vi "Event 練習-五子棋-介面.vi"() -> ()   [LabVIEW 2019, in "Event 2-上課練習.lvlib"]
uses:
  <vilib>/Utility/miscctls.llb/LVPoint32TypeDef.ctl
panel:
  out "Coords":T1
  out "黑子":T2[][](array[typedef])
  out "白子":T3[][](array[typedef])
  in  "stop":bool
  # "五子棋程式-1（練習Event搭配State Machine的結構)\n1. 練習如何建立棋盤、黑子、白子；\n2. 按下「半黑白」可產生上下各一半的棋子，再按一次清除；\n3. 在滑鼠按下處，產生黑子；再按一次可以消除；"
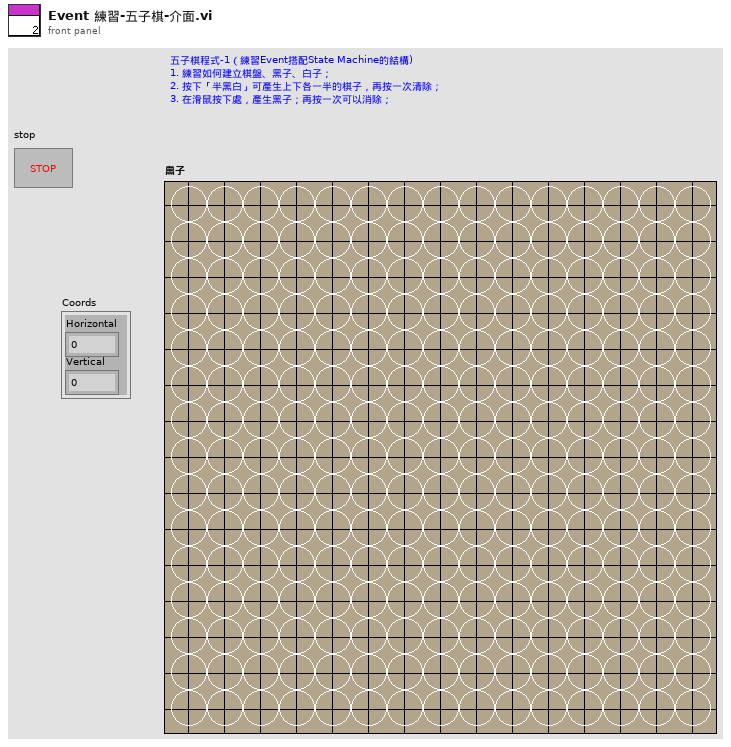
[diagram p1: front panel]
types:
  T1 = typedef "LVPoint32TypeDef.ctl" = cluster{"Horizontal":i32, "Vertical":i32}
  T2 = typedef "Event 2-上課練習.lvlib/黑子.ctl" = bool
  T3 = typedef "Event 2-上課練習.lvlib/白子.ctl" = bool
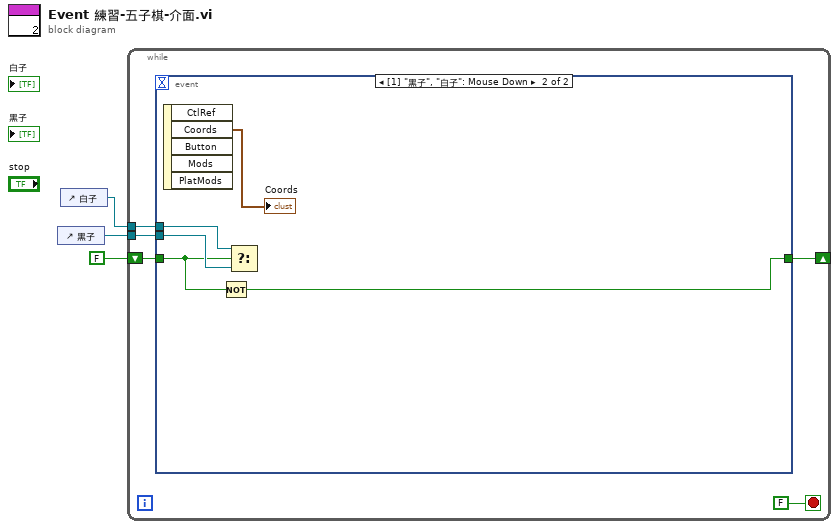
[diagram p0: block diagram]
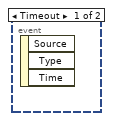
[diagram p2: hidden frame]
diagram:
  n1 = control-ref of="黑子"() -> (w2:refnum<vi>)
  n2 = control-ref of="白子"() -> (w1:refnum<vi>)
  n3 = while {
    shift-right: [w4] -> _
    shift-left: FALSE -> [w7]
    tunnel: w2 -> [w6]
    tunnel: w1 -> [w5]
    stop <- FALSE stop-if-true
    n4 = event shown="[1] \"黑子\", \"白子\": Mouse Down" {
      selector: _ -> [_ _]
      dyn-events: _ -> [_ _]
      timeout: _ -> [_ _]
      tunnel: w7 -> [_ w10]
      tunnel: w6 -> [_ w12]
      tunnel: w5 -> [_ w11]
      tunnel: [_ w9] -> w4
      event Timeout {
        n5 = event-data() -> ()  [unwired: 1 in, 3 out]
      }
      event "黑子", "白子": Mouse Down {
        n6 = event-data() -> ("Coords"=→"Coords":T1)  [unwired: 1 in, 4 out]
        n7 = Not(x=w10) -> (.not. x?=w9:bool)
        n8 = Select(t=w11, s=w10, f=w12) -> ()  [unwired: 1 out]
      }
    }
  }
